vi "Get Images Array.vi"(11 "Error In":errorcluster) -> (4 "Ref Array":T1[](array[typedef]), 8 "Names":string[](array[string]), 15 "Error Out":errorcluster)   [LabVIEW 2020]
uses:
  <vilib>/vision/Image Controls.llb/IMAQ Image.ctl
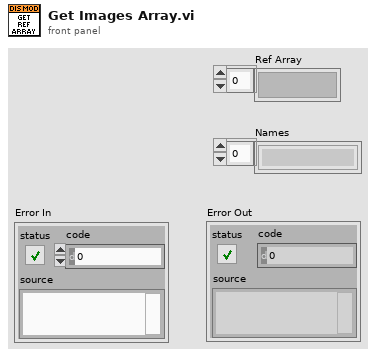
[diagram p1: front panel]
types:
  T1 = typedef "IMAQ Image.ctl" = refnum<image>
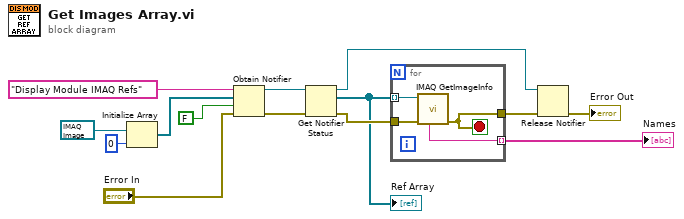
[diagram p0: block diagram]
diagram:
  n1 = Initialize Array(T1 refnum ("New Image"), 0 ("dimension size")) -> (w10:T1[])
  n2 = Obtain Notifier(name (unnamed)="Display Module IMAQ Refs", notification data type=w10, create if not found? (T)=FALSE, error in (no error)="Error In") -> (notifier out=w8:refnum<notifier>, error out=w7:errorcluster)  [unwired: 1 out]
  n3 = Get Notifier Status(notifier=w8, error in (no error)=w7) -> (notifier out=w3:refnum<notifier>, current notification=w2:T1[], error out=w5:errorcluster)  [unwired: 2 out]
  "Ref Array" <- w2
  n4 = for {
    tunnel: w2 -> [w18] mode=indexing
    tunnel: [w17] -> w1 mode=indexing
    tunnel: w5 -> [w16]
    tunnel: [w15] -> w4
    stop <- w15 stop-if-true
    n5 = call "IMAQ GetImageInfo"("error in (no error)"=w16, "Image"=w18) -> ("error out"=w15:errorcluster, "Image Name"=w17:string)  [unwired: 2 in, 6 out]
  }
  "Names" <- w1
  n6 = Release Notifier(notifier=w3, error in (no error)=w4) -> (error out=→"Error Out":errorcluster)  [unwired: 1 in, 2 out]
